vi "InstrQuery.vi"(8 "error in (no error)":errorcluster, 10 "Command string":string, 11 "InstControl in":refnum<class "InstrControl.lvclass">) -> (0 "error out":errorcluster, 2 "Instrument response":string, 3 "InstControl out":refnum<class "InstrControl.lvclass">)   [LabVIEW 2019, in "InstrControl.lvclass"]
uses:
  InstrControl.lvclass
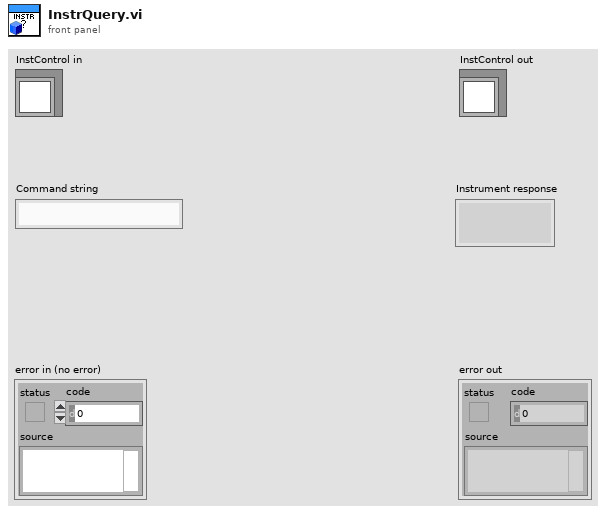
[diagram p1: front panel]
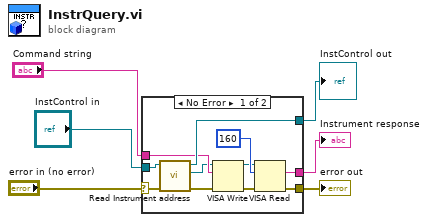
[diagram p0: block diagram]
diagram:
  n1 = case shown="No Error" "error in (no error)" {
    selector: "error in (no error)" -> [w16 w19]
    tunnel: [w7 w19] -> w5
    tunnel: [w15 w18] -> w3
    tunnel: "InstControl in" -> [w17 w18]
    tunnel: "Command string" -> [w11 _]
    tunnel: [w10 _] -> w1
    frame No Error {
      n2 = call-dynamic "Read Instrument address.vi"("error in (no error)"=w16, "InstControl in"=w17) -> ("error out"=w9:errorcluster, "GPIB address"=w8:refnum<visa-resource-name>, "InstControl out"=w15:refnum<class "InstrControl.lvclass">)  [unwired: 7 in]
      n3 = VISA Write(VISA resource name=w8, write buffer=w11, error in (no error)=w9) -> (VISA resource name out=w13:refnum<visa-resource-name>, error out=w12:errorcluster)  [unwired: 1 out]
      n4 = VISA Read(VISA resource name=w13, byte count=160, error in (no error)=w12) -> (read buffer=w10:string, error out=w7:errorcluster)  [unwired: 2 out]
    }
    frame Error {
    }
  }
  "error out" <- w5
  "InstControl out" <- w3
  "Instrument response" <- w1
